vi "TEST_bench_FXP_A_times_x_iterate_32bit.vi"(6 "NS + 1":u8=9) -> ()   [LabVIEW 2017]
uses:
  fixed-point/typeDefs/UT_matrix_data.ctl
  fixed-point/typeDefs/Bz_vec_scalar.ctl
  fixed-point/typeDefs/Lz_vec_scalar.ctl
  fixed-point/typeDefs/Kz_vec_scalar.ctl
  fixed-point/typeDefs/Nx_vec_scalar.ctl
  fixed-point/typeDefs/Az_vec_scalar.ctl
  fixed-point/typeDefs/x_vec_scalar.ctl
  fixed-point/typeDefs/Cz_vec_scalar.ctl
  fixed-point/typeDefs/x_vec_bram.ctl
  fixed-point/typeDefs/A_as_vec_bram.ctl
  <vilib>/rvi/DataTransferAndStorage/Container/Common/niFpgaContainerExecOnDevCompGetState.vi
  <vilib>/rvi/Emulation/niFpgaEmulationIsFPGAContextNoSignature.vi
  <vilib>/rvi/DataTransferAndStorage/Container/Common/niFpgaContainerGetUniqueNameForEmu.vi
  <vilib>/rvi/Emulation/niFpgaProcessEmulError.vi
  <vilib>/rvi/Emulation/niFpgaSctlEmulationGetInTimedLoop.vi
  <vilib>/rvi/errors/nirviReportUnexpectedCaseInternalError (U32).vi
  <vilib>/rvi/Memory/Memory_Emulation/niFpgaMemoryEmulationCacheClearOnFirstRun.vi
  <vilib>/rvi/Memory/Memory_Emulation/nirvimemoryEmulationManagerCache_MakeExclusive.vi
  <vilib>/rvi/Memory/Memory_Emulation/niFpgaMemoryEmulationValidateCache.vi
  <vilib>/rvi/Memory/Memory_Emulation/nirvimemoryEmulationManagerCache_InsertValue.vi
  <vilib>/Utility/error.llb/Clear Errors.vi
  <vilib>/rvi/Memory/Memory_Emulation/nirvimemoryEmulationManagerCache_ReleaseExclusive.vi
  <vilib>/rvi/Memory/Memory_Emulation/nirvimemoryEmulationManagerCache_GetValue.vi
  <vilib>/rvi/Memory/Memory_Emulation/nirvimemoryEmulationManagerCache_SetValue.vi
  <vilib>/rvi/Emulation/niFpgaSctlEmulationResourceMgr.vi
  <vilib>/rvi/DataTransferAndStorage/Container/XNode/niFpgaContainer.xnode
  <vilib>/rvi/Memory/Memory_Emulation/niFpgaMemoryEmulationRefIn.vi
panel:
  out "xk_1_1":fxp<+/-,32,6>[](array[numeric])
  out "A*x":fxp<+/-,32,13>[](array[numeric])
  in  "NumIter":i32
  in  "matrix data":T1
  out "Y":fxp<+/-,32,6>[](array[numeric])
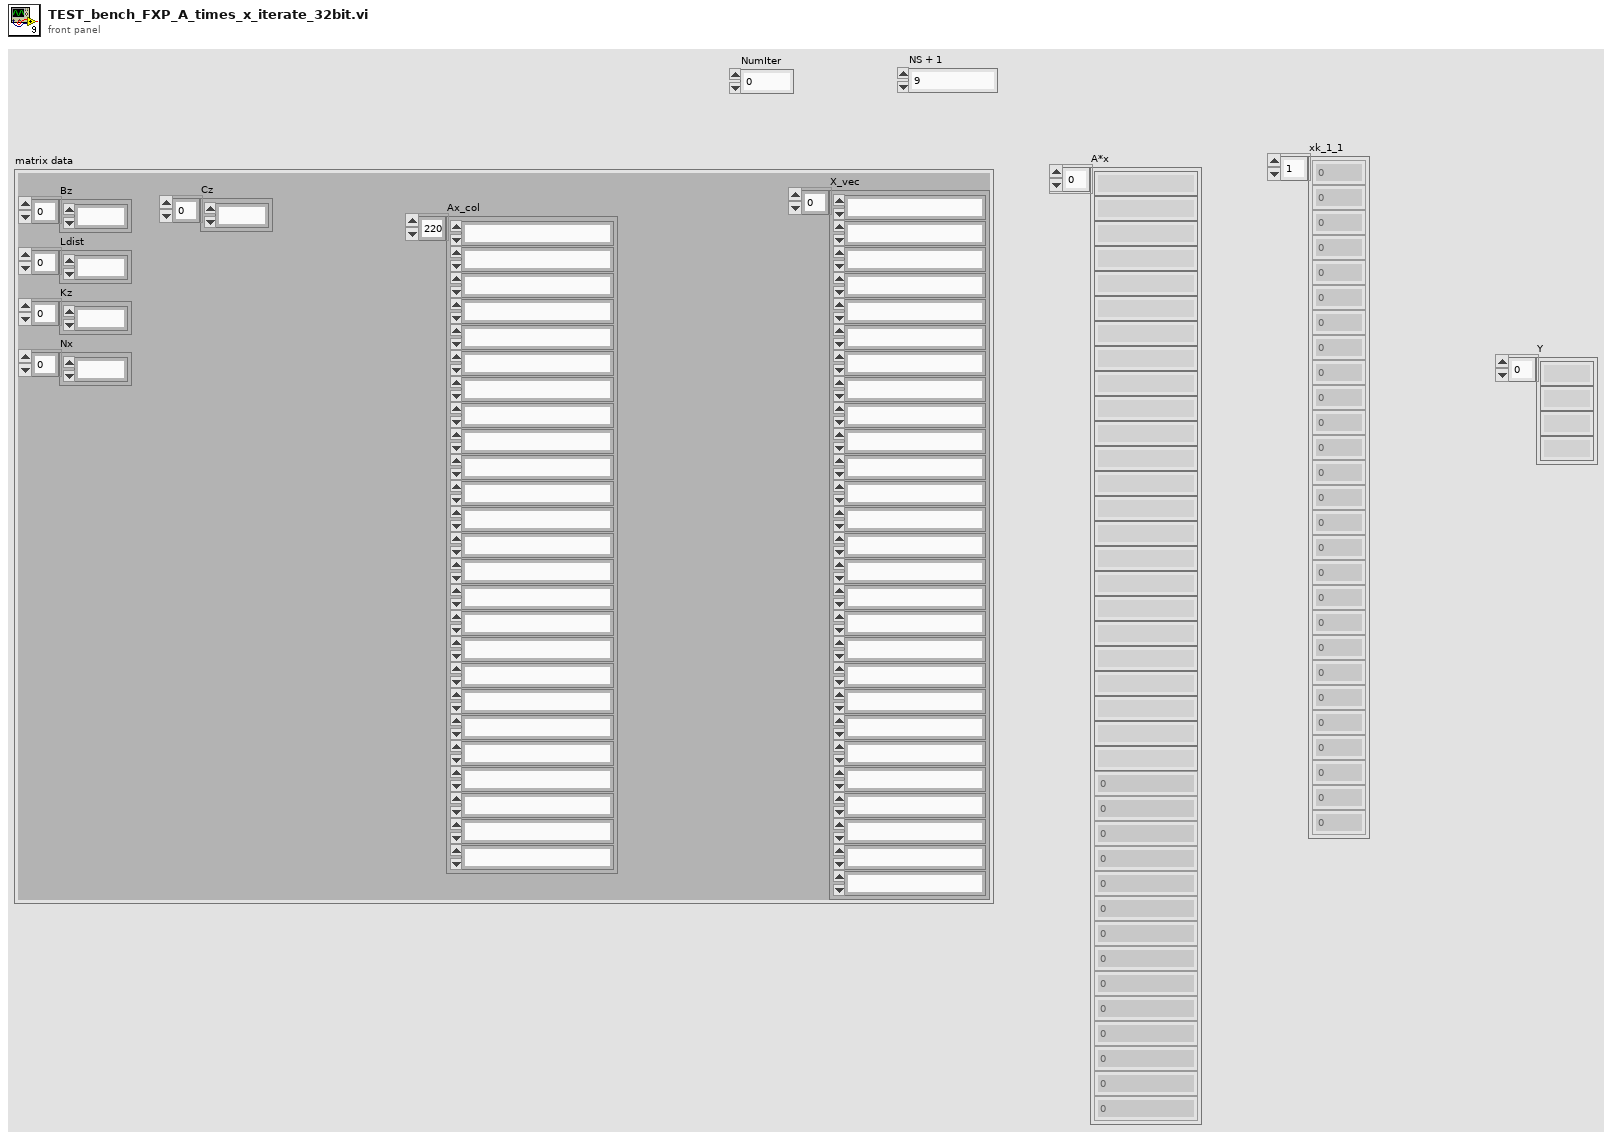
[diagram p1: front panel]
types:
  T1 = typedef "UT_matrix_data.ctl" = cluster{"Bz":T2[], "Ldist":T3[], "Kz":T4[], "Nx":T5[], "Ax_col":T6[], "X_vec":T7[], "Cz":T8[]}
  T2 = typedef "Bz_vec_scalar.ctl" = fxp<+/-,32,3>
  T3 = typedef "Lz_vec_scalar.ctl" = fxp<+/-,32,3>
  T4 = typedef "Kz_vec_scalar.ctl" = fxp<+/-,32,10>
  T5 = typedef "Nx_vec_scalar.ctl" = fxp<+/-,32,2>
  T6 = typedef "Az_vec_scalar.ctl" = fxp<+/-,32,7>
  T7 = typedef "x_vec_scalar.ctl" = fxp<+/-,32,6>
  T8 = typedef "Cz_vec_scalar.ctl" = fxp<+/-,32,4>
  T9 = typedef "x_vec_bram.ctl" = refnum<k21>
  T10 = typedef "A_as_vec_bram.ctl" = refnum<k21>
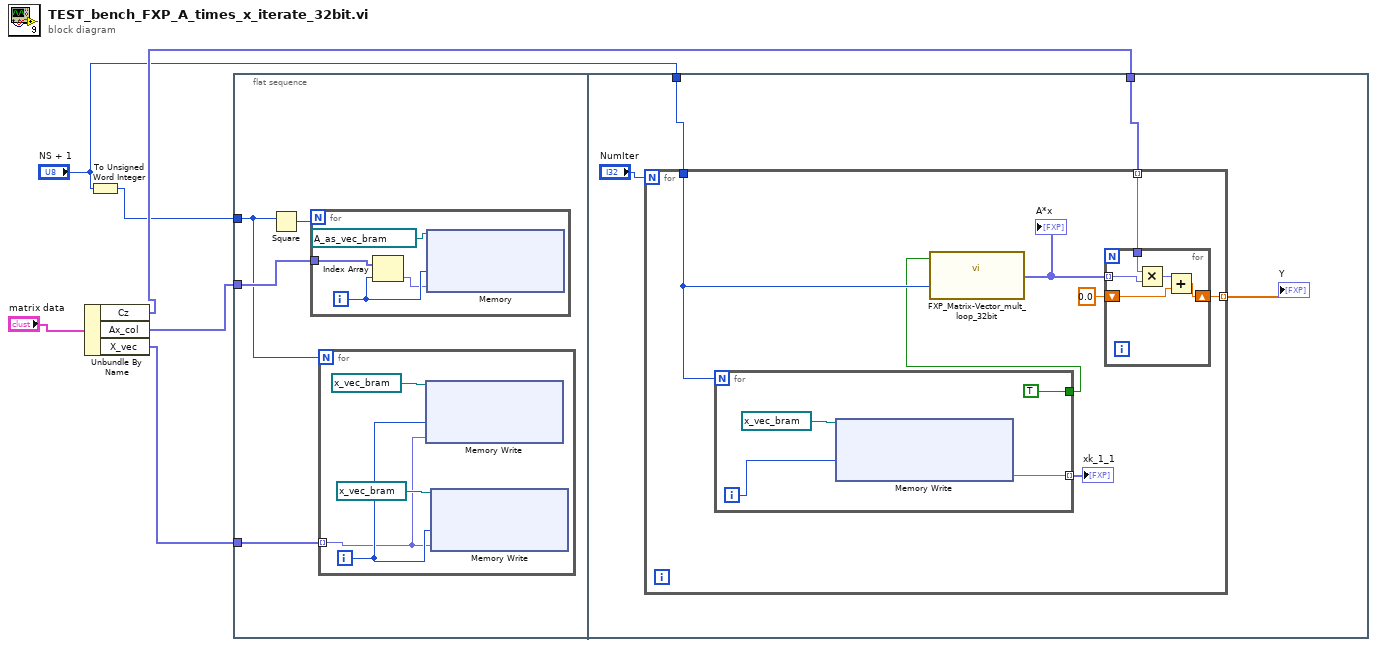
[diagram p0: block diagram]
diagram:
  n1 = Unbundle By Name("matrix data") -> ("Cz"=w3:T8[], "Ax_col"=w5:T6[], "X_vec"=w4:T7[])
  n2 = To Unsigned Word Integer(number="NS + 1") -> (unsigned 16bit integer=w1:u16)
  n3 = flat-sequence {
    tunnel: w1 -> [w7]
    tunnel: w5 -> [w10]
    tunnel: w4 -> [w9]
    tunnel: "NS + 1" -> [w22]
    tunnel: w3 -> [w21]
    frame #0 {
      n4 = Square(x=w7) -> (x^2=w8:u16)
      n5 = for {
        N: w8 -> [_]
        tunnel: w10 -> [w17]
        i -> [w16]
        n6 = Index Array(array=w17, index=w16) -> (element=w15:T6)
        n7 = xnode "Memory"("Address"=w16, "Data"=w15, "Memory In"=T10 "AasCol _FXP") -> ()  [unwired: 1 out]
      }
      n8 = for {
        N: w7 -> [_]
        tunnel: w9 -> [w11] mode=indexing
        i -> [w12]
        n9 = xnode "Memory Write"("Address"=w12, "Data"=w11, "Memory In"=T9 "xk_1_1" ("Memory")) -> ()  [unwired: 1 out]
        n10 = xnode "Memory Write"("Address"=w12, "Data"=w11, "Memory In"=T9 "xk_1_0" ("Memory")) -> ()  [unwired: 1 out]
      }
    }
    frame #1 {
      n11 = for {
        N: "NumIter" -> [_]
        tunnel: w22 -> [w25]
        tunnel: w21 -> [w28] mode=indexing
        tunnel: [w26] -> w20 mode=indexing
        n12 = for {
          N: w25 -> [_]
          tunnel: [w31] -> w24 mode=indexing
          tunnel: [TRUE] -> w23
          i -> [w32]
          n13 = xnode "Memory Write"("Address"=w32, "Memory In"=T9 "xk_1_1" ("Memory")) -> ("Data"=w31:fxp<+/-,32,6>)  [unwired: 1 out]
        }
        "xk_1_1" <- w24
        n14 = call "FXP_Matrix-Vector_mult_loop_32bit.vi"("Ns_2"=w25, "inputValid"=w23) -> ("Array"=w29:fxp<+/-,32,13>[])  [unwired: 9 in]
        "A*x" <- w29
        n15 = for {
          tunnel: w29 -> [w37] mode=indexing
          tunnel: w28 -> [w38]
          shift-right: [w35] -> w26
          shift-left: sgl 0.0 -> [w34]
          n16 = Multiply(x=w38, y=w37) -> (x*y=w36:fxp<+/-,64,17>)
          n17 = Add(x=w36, y=w34) -> (x+y=w35:sgl)
        }
      }
      "Y" <- w20
    }
  }
